vi "InitQueues.vi"(8 "error in (no error)":errorcluster, 11 "Stream in":refnum<class "Stream.lvclass">) -> (0 "error out":errorcluster, 3 "Stream out":refnum<class "Stream.lvclass">)   [LabVIEW 2018, in "Stream.lvclass"]
uses:
  Stream.lvclass
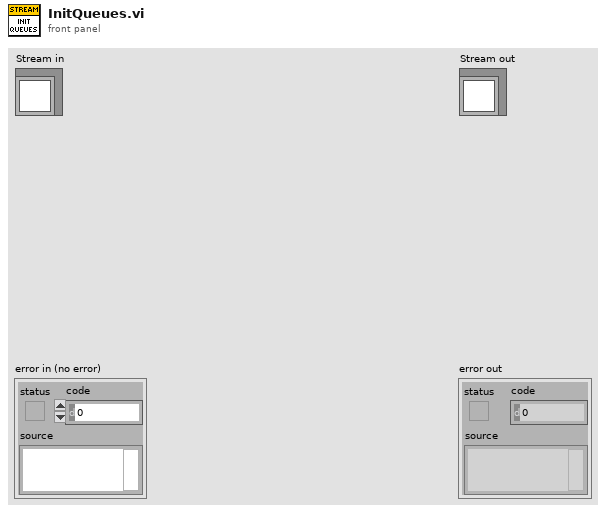
[diagram p1: front panel]
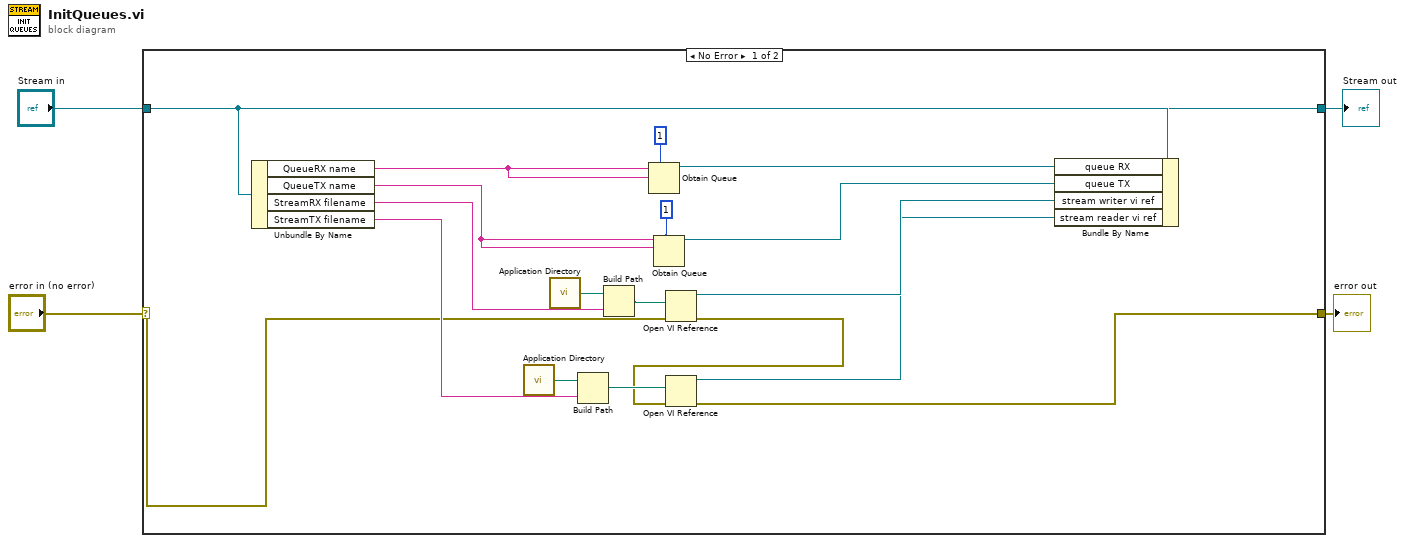
[diagram p0: block diagram]
diagram:
  n1 = case shown="No Error" "error in (no error)" {
    selector: "error in (no error)" -> [w9 w25]
    tunnel: [w5 w25] -> w3
    tunnel: [w16 w24] -> w1
    tunnel: "Stream in" -> [w17 w24]
    frame No Error {
      n2 = Unbundle By Name(w17) -> ("QueueRX name"=w19:string, "QueueTX name"=w18:string, "StreamRX filename"=w11:string, "StreamTX filename"=w10:string)
      n3 = call <vilib>:"Application Directory.vi"() -> ("Application Directory"=w13:path)
      n4 = call <vilib>:"Application Directory.vi"() -> ("Application Directory"=w14:path)
      n5 = Build Path(base path=w13, name or relative path=w10) -> (appended path=w12:path)
      n6 = Build Path(base path=w14, name or relative path=w11) -> (appended path=w15:path)
      n7 = Obtain Queue(max queue size (-1, unlimited)=1, name (unnamed)=w19, element data type=w19) -> (queue out=w20:refnum<queue>)  [unwired: 2 in, 2 out]
      n8 = Obtain Queue(max queue size (-1, unlimited)=1, name (unnamed)=w18, element data type=w18) -> (queue out=w21:refnum<queue>)  [unwired: 2 in, 2 out]
      n9 = Open VI Reference(vi path=w15, error in (no error)=w9) -> (vi reference=w8:refnum<vi>, error out=w7:errorcluster)  [unwired: 4 in]
      n10 = Open VI Reference(vi path=w12, error in (no error)=w7) -> (vi reference=w6:refnum<vi>, error out=w5:errorcluster)  [unwired: 4 in]
      n11 = Bundle By Name(cluster=w17, "queue RX"=w20, "queue TX"=w21, "stream writer vi ref"=w8, "stream reader vi ref"=w6) -> (w16:refnum<class "Stream.lvclass">)
    }
    frame Error {
    }
  }
  "error out" <- w3
  "Stream out" <- w1
